vi "LWXPS_GroupVelocityCurrentGet.vi"(0 "XPS Reference IN":refnum<k24>, 5 "Group Name":string, 7 "Number of positioners":i32, 11 "LabVIEW error IN":errorcluster) -> (4 "XPS Reference OUT":refnum<k24>, 6 "Returned error code":i32, 8 "Current Velocity":dbl[](array[numeric]), 10 "XPS Error String":string, 15 "LabVIEW error OUT":errorcluster)   [LabVIEW 2014]
uses:
  D:/XPSQ8_LabView_Library/Development/Source/Dll/Newport.XPS.CommandInterface.dll
  Dll/Newport.XPS.CommandInterface.dll
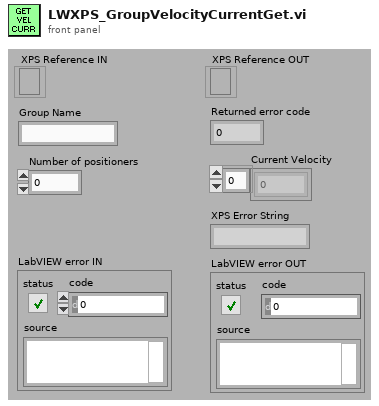
[diagram p1: front panel]
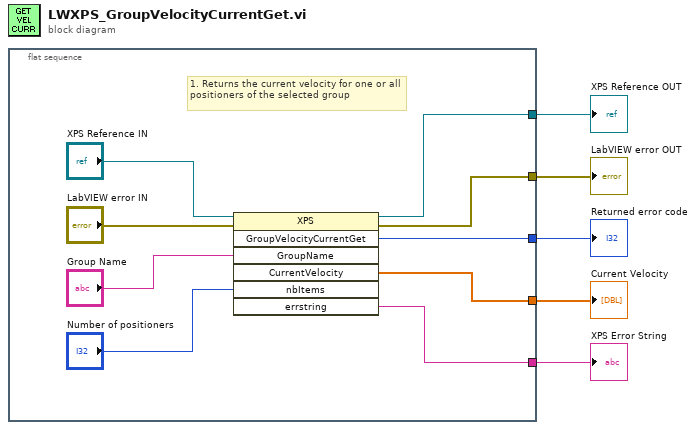
[diagram p0: block diagram]
diagram:
  n1 = flat-sequence {
    tunnel: [w10] -> w5
    tunnel: [w12] -> w4
    tunnel: [w13] -> w3
    tunnel: [w9] -> w1
    tunnel: [w8] -> w2
    frame #0 {
      # "1. Returns the current velocity for one or all positioners of the selected group"
      n2 = invoke class="XPS" method="GroupVelocityCurrentGet"(reference="XPS Reference IN", error in="LabVIEW error IN", "GroupName"="Group Name", "nbItems"="Number of positioners") -> (reference out=w10:refnum<k24>, error out=w12:errorcluster, "GroupVelocityCurrentGet"=w13:i32, "CurrentVelocity"=w9:dbl[], "errstring"=w8:string)  [unwired: 3 in, 2 out]
    }
  }
  "XPS Reference OUT" <- w5
  "LabVIEW error OUT" <- w4
  "Returned error code" <- w3
  "XPS Error String" <- w2
  "Current Velocity" <- w1
